vi "Ref_3.vi"(0 "Trip  Ch 1":refnum<vi>, 1 "Trip  Ch 2":refnum<vi>, 3 "Trip  Ch 3":refnum<vi>, 4 "Trip  Ch 4":refnum<vi>, 5 "Trip  Ch 5":refnum<vi>, 7 "Trip  Ch 6":refnum<vi>, 8 "Trip  Ch 7":refnum<vi>, 9 "Trip  Ch 8":refnum<vi>, 10 "Init_F":bool=TRUE, 12 "Trip  Ch 9":refnum<vi>, 13 "Trip  Ch 10":refnum<vi>) -> (14 "Trip  Ch 1 out":refnum<vi>, 15 "Trip  Ch 2 out":refnum<vi>, 16 "Trip  Ch 3 out":refnum<vi>, 17 "Trip  Ch 4 out":refnum<vi>, 19 "Trip  Ch 5 out":refnum<vi>, 20 "Trip  Ch 6 out":refnum<vi>, 21 "Trip  Ch 7 out":refnum<vi>, 23 "Trip  Ch 8 out":refnum<vi>, 24 "Trip  Ch 9 out":refnum<vi>, 25 "Trip  Ch 10 out":refnum<vi>)   [LabVIEW 2017]
panel:
  out "error out":errorcluster
  in  "error in":errorcluster
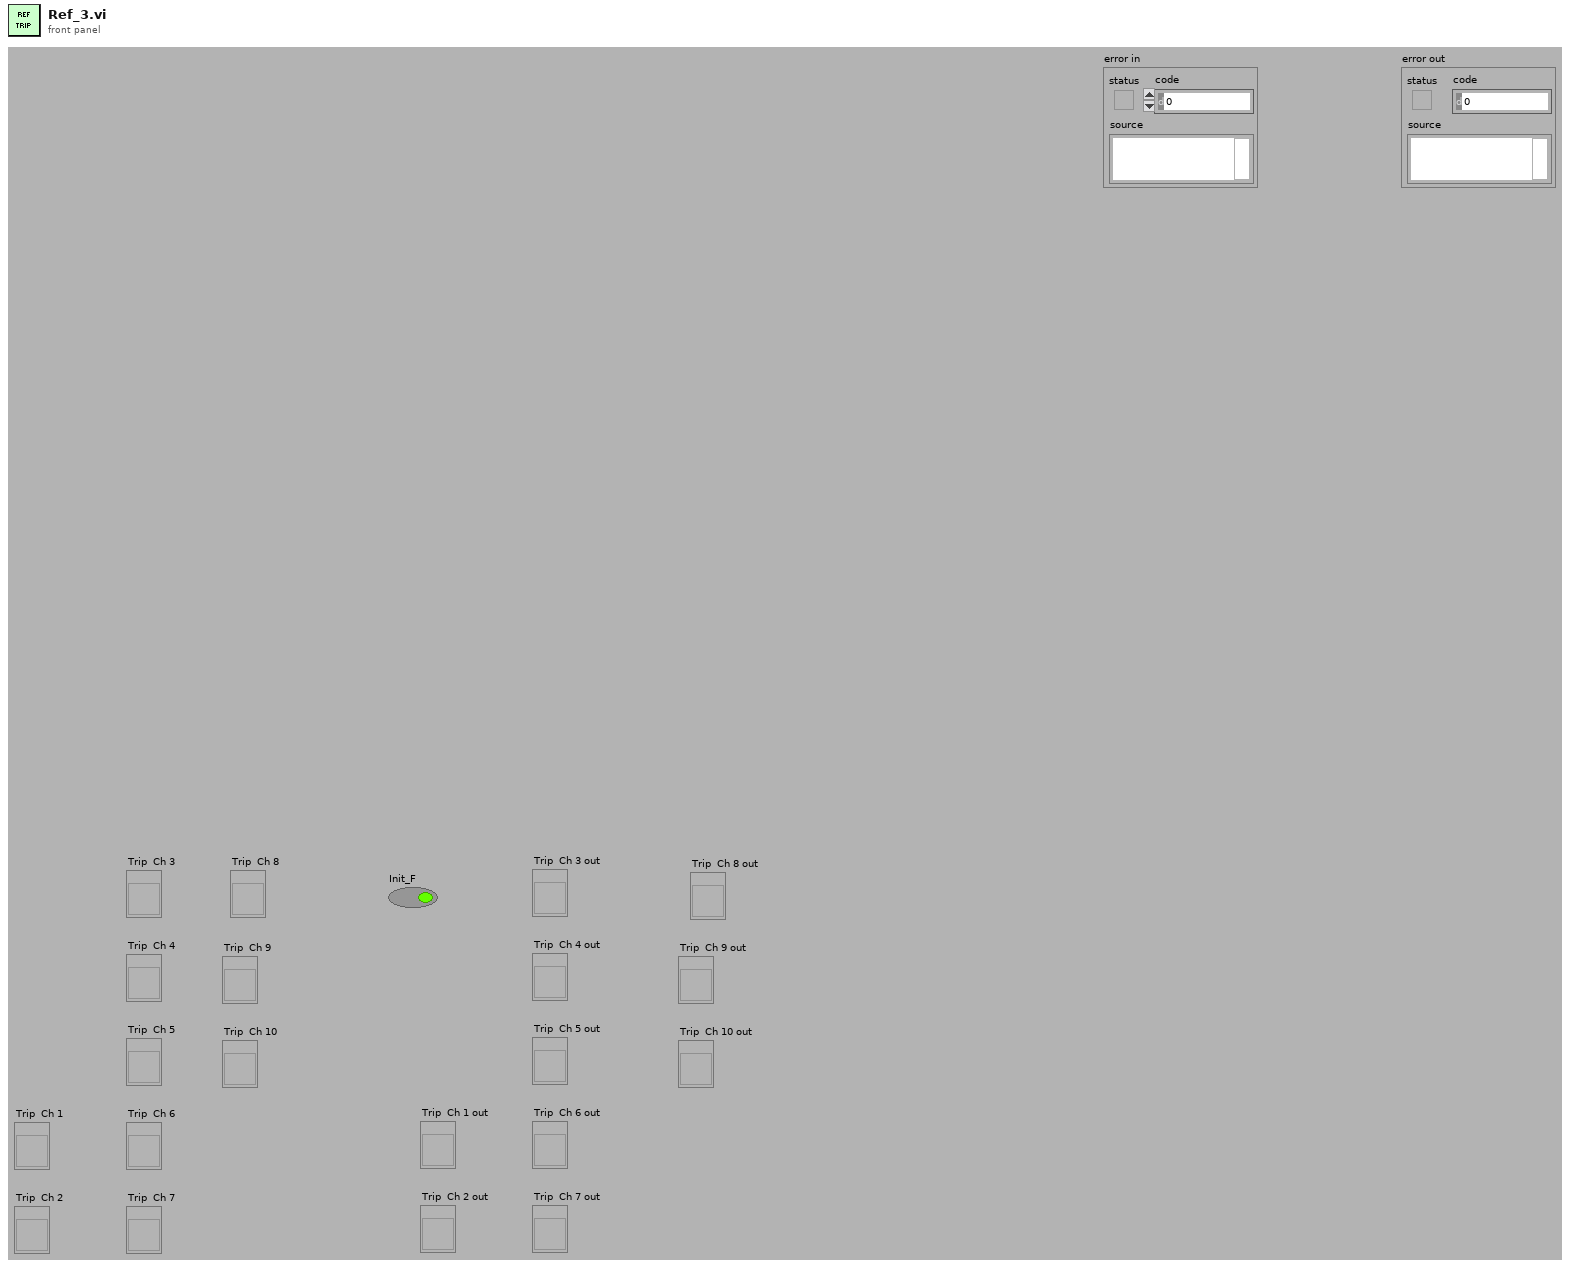
[diagram p1: front panel]
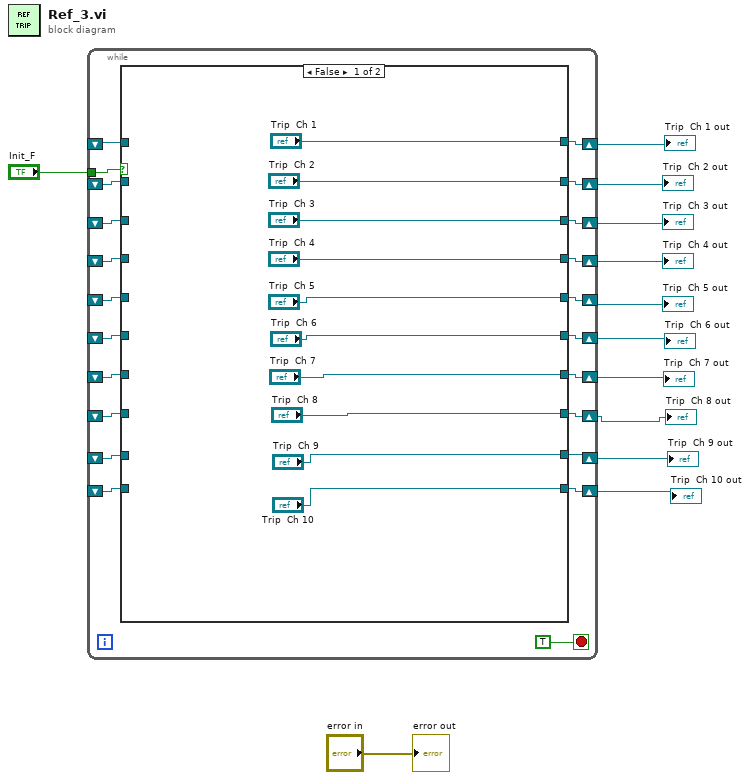
[diagram p0: block diagram]
diagram:
  n1 = while {
    shift-right: [w33] -> w4
    shift-left: _ -> [w32]
    tunnel: "Init_F" -> [w31]
    shift-right: [w30] -> w5
    shift-left: _ -> [w23]
    shift-right: [w29] -> w6
    shift-left: _ -> [w22]
    shift-right: [w28] -> w7
    shift-left: _ -> [w17]
    shift-right: [w27] -> w8
    shift-left: _ -> [w21]
    shift-right: [w26] -> w9
    shift-left: _ -> [w20]
    shift-right: [w25] -> w10
    shift-left: _ -> [w19]
    shift-right: [w24] -> w1
    shift-left: _ -> [w18]
    shift-right: [w16] -> w3
    shift-left: _ -> [w14]
    shift-right: [w15] -> w2
    shift-left: _ -> [w13]
    stop <- TRUE stop-if-true
    n2 = case shown="False" w31 {
      tunnel: ["Trip  Ch 1" w54] -> w33
      tunnel: w32 -> [_ w54]
      tunnel: ["Trip  Ch 2" w47] -> w30
      tunnel: ["Trip  Ch 3" w48] -> w29
      tunnel: ["Trip  Ch 4" w49] -> w28
      tunnel: ["Trip  Ch 5" w50] -> w27
      tunnel: ["Trip  Ch 6" w51] -> w26
      tunnel: ["Trip  Ch 7" w52] -> w25
      tunnel: ["Trip  Ch 8" w53] -> w24
      tunnel: w23 -> [_ w47]
      tunnel: w22 -> [_ w48]
      tunnel: w21 -> [_ w50]
      tunnel: w20 -> [_ w51]
      tunnel: w19 -> [_ w52]
      tunnel: w18 -> [_ w53]
      tunnel: w17 -> [_ w49]
      tunnel: ["Trip  Ch 9" w46] -> w16
      tunnel: ["Trip  Ch 10" w45] -> w15
      tunnel: w14 -> [_ w46]
      tunnel: w13 -> [_ w45]
      frame False {
      }
      frame True {
      }
    }
  }
  "Trip  Ch 8 out" <- w1
  "Trip  Ch 7 out" <- w10
  "Trip  Ch 6 out" <- w9
  "Trip  Ch 5 out" <- w8
  "Trip  Ch 4 out" <- w7
  "Trip  Ch 3 out" <- w6
  "Trip  Ch 2 out" <- w5
  "Trip  Ch 1 out" <- w4
  "Trip  Ch 9 out" <- w3
  "Trip  Ch 10 out" <- w2
  "error out" <- "error in"
